vi "gfitsio-write-column-sgl-scalar.vi"(4 "units":string, 6 "row":i32, 7 "column":string, 8 "error in (no error)":errorcluster, 9 "data":sgl, 11 "gfits refnum":T1) -> (0 "error out":errorcluster, 3 "dup gfits refnum":T1)   [LabVIEW 2011, in "gfitsio.lvlib"]
doc: "Write data to the table column (doing data type conversion if necessary)."
uses:
  gfitsio.lvlib
  gfitsio-refnum.ctl
  cfitsio-hdutypes.ctl
  gfitsio.dll
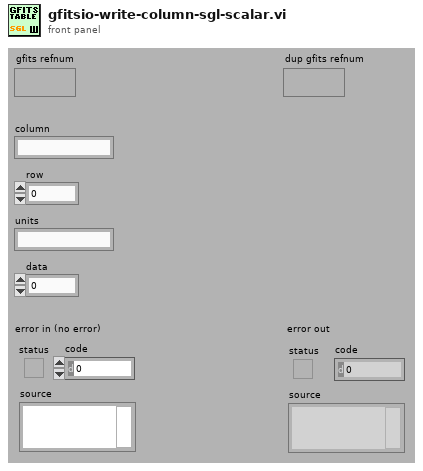
[diagram p1: front panel]
types:
  T1 = typedef "gfitsio.lvlib/gfitsio-refnum.ctl" = refnum<k1>
  T2 = typedef "gfitsio.lvlib/cfitsio-hdutypes.ctl" = i32
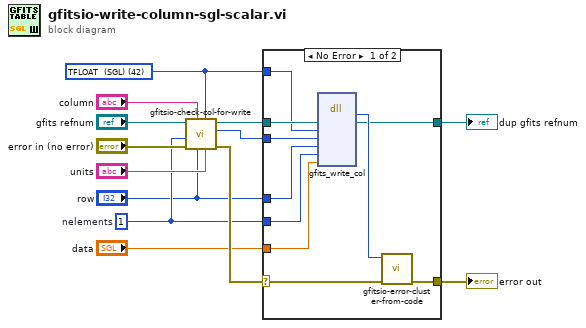
[diagram p0: block diagram]
diagram:
  w2 = T2 42 items=["TBIT"=1, "TBYTE  (U8)"=11, "TSBYTE  (I8)"=12, "TLOGICAL"=14, "TSTRING"=16, "TUSHORT  (U16)"=20, "TSHORT  (I16)"=21, "TUINT"=31, "TULONG  (U32)"=40, "TLONG  (I32)"=41, "TFLOAT  (SGL)"=42, "TLONGLONG  (I64)"=81, "TDOUBLE"=82, "TCOMPLEX  (CSG)"=83, "TDOUBLECOMPLEX  (CDB)"=163] ("cfitsio datatype")
  w3 = 1  # nelements
  n1 = call "gfitsio-check-col-for-write.vi"("units"="units", "cfitsio datatype"=w2, "row"="row", "column"="column", "error in (no error)"="error in (no error)", "size (-1:variable)"=w3, "gfits refnum"="gfits refnum") -> ("error out"=w8:errorcluster, "colnum"=w5:i32, "dup gfits refnum"=w10:T1)  [unwired: 2 in]
  n2 = case shown="No Error" w8 {
    selector: w8 -> [w23 w25]
    tunnel: [w22 w25] -> w12
    tunnel: w10 -> [w19 w24]
    tunnel: [w20 w24] -> w13
    tunnel: w5 -> [w18 _]
    tunnel: w2 -> [w17 _]
    tunnel: "row" -> [w16 _]
    tunnel: "data" -> [w15 _]
    tunnel: w3 -> [w14 _]
    frame No Error {
      n3 = dll-call lib="C:/BonOMM/BonOMM-SAOMM/SubVIs/gfitsio/gfitsio.dll" fn="gfits_write_col"("dup gfits refnum"=w19, "datatype"=w17, "column"=w18, "row"=w16, "nelements"=w14, "data"=w15) -> (w21:i32, "dup gfits refnum"=w20:T1)  [unwired: 8 in, 2 out]
      n4 = call "gfitsio-error-cluster-from-code.vi"("error in (no error)"=w23, "error code"=w21) -> ("error out"=w22:errorcluster)  [unwired: 9 in]
    }
    frame Error {
    }
  }
  "error out" <- w12
  "dup gfits refnum" <- w13
